vi "Generuj_Error.vi"(6 "Generuj (F)":bool, 8 "Generator":errorcluster, 11 "error in (no error)":errorcluster) -> (3 "error out":errorcluster)   [LabVIEW 2013]
doc: "Generuje zadany błąd lub ostrzeżenie"
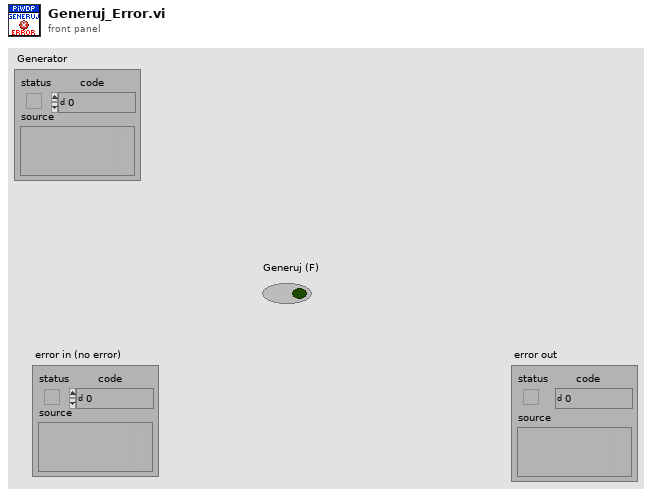
[diagram p1: front panel]
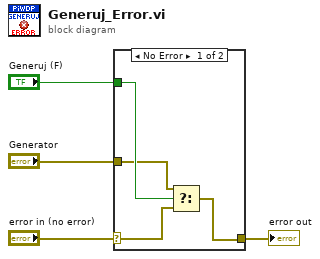
[diagram p0: block diagram]
diagram:
  n1 = case shown="No Error" "error in (no error)" {
    selector: "error in (no error)" -> [w6 w9]
    tunnel: [w5 w9] -> w3
    tunnel: "Generator" -> [w7 _]
    tunnel: "Generuj (F)" -> [w8 _]
    frame No Error {
      n2 = Select(t=w7, s=w8, f=w6) -> (s? t:f=w5:errorcluster)
    }
    frame Error {
    }
  }
  "error out" <- w3
